vi "Finish.vi"   [LabVIEW 2013]
doc: "This VI is called just before exiting. It is expected to close I/O refnum, save collected data, etc."
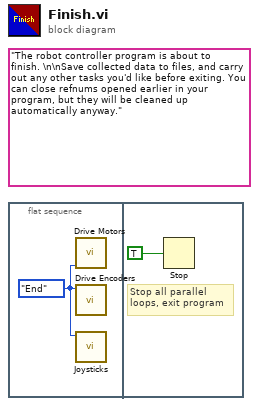
[diagram p0: block diagram]
diagram:
  (unwired) "The robot controller program is about to finish. \n\nSave collected data to files, and carry out any other tasks you'd like before exiting. You can close refnums opened earlier in your program, but they will be cleaned up automatically anyway."
  n1 = flat-sequence {
    frame #0 {
      w1 = enum16{"Init", "Run", "End"}."End" ("Mode")
      n2 = call "Drive Motors.vi"("Mode"=w1) -> ()  [unwired: 2 in, 9 out]
      n3 = call "Drive Encoders.vi"("Mode"=w1) -> ()  [unwired: 3 in, 8 out]
      n4 = call "Joysticks.vi"("Mode"=w1) -> ()  [unwired: 9 out]
    }
    frame #1 {
      # "Stop all parallel\nloops, exit program"
      n5 = Stop(stop? (T)=TRUE ("Quit")) -> ()
    }
  }
